vi "IMURead.vi"(0 "AdaIMUDevRef":T4={"DevStatus"={"status"=FALSE, "code"=0, "source"=""}, "Gyro Address"=0, "Gyro Range"=0, "Mean Rates"={"Xmo"=0.0, "Ymo"=0.0, "Zmo"=0.0}, "StdDev Rates"={"Xsdo"=0.0, "Ysdo"=0.0, "Zsdo"=0.0}, "Fast"=FALSE, "Reset"=FALSE, "Accel Address"=0, "Accel Range"=0, "Accel Scale"={"Xscale"=0.0, "Yscale"=0.0, "Zscale"=0.0}, "Mag Address"=0, "Mag Range"=0, "G Sense"=FALSE, "A Sense"=FALSE, "M Sense"=FALSE, "Accel Offset"={"Xzero"=0.0, "Yzero"=0.0, "Zzero"=0.0}, "Motion Thresh"=0.0, "Mag Scale"={"Xscale"=1.0, "Yscale"=1.0, "Zscale"=1.0}, "Mag Offset"={"Xzero"=1.0, "Yzero"=1.0, "Zzero"=1.0}, "I2C Bus"=enum."I2C On-Board", "Handle"=0, "Anomaly Thresh"=0.0, "Local Mag"=0.0}, 11 "error in":errorcluster) -> (4 "AdaIMUDevRef Out":T4={"DevStatus"={"status"=FALSE, "code"=0, "source"=""}, "Gyro Address"=0, "Gyro Range"=0, "Mean Rates"={"Xmo"=0.0, "Ymo"=0.0, "Zmo"=0.0}, "StdDev Rates"={"Xsdo"=0.0, "Ysdo"=0.0, "Zsdo"=0.0}, "Fast"=FALSE, "Reset"=FALSE, "Accel Address"=0, "Accel Range"=0, "Accel Scale"={"Xscale"=0.0, "Yscale"=0.0, "Zscale"=0.0}, "Mag Address"=0, "Mag Range"=0, "G Sense"=FALSE, "A Sense"=FALSE, "M Sense"=FALSE, "Accel Offset"={"Xzero"=0.0, "Yzero"=0.0, "Zzero"=0.0}, "Motion Thresh"=0.0, "Mag Scale"={"Xscale"=1.0, "Yscale"=1.0, "Zscale"=1.0}, "Mag Offset"={"Xzero"=1.0, "Yzero"=1.0, "Zzero"=1.0}, "I2C Bus"=enum."I2C On-Board", "Handle"=0, "Anomaly Thresh"=0.0, "Local Mag"=0.0}, 6 "Gyro":T3, 8 "Accel":T1={"Xaccel"=0.0, "Yaccel"=0.0, "Zaccel"=0.0, "Motion"=FALSE, "Threshold"=0.04, "FreeFall"=FALSE}, 10 "Mag":T2, 15 "error out":errorcluster)   [LabVIEW 2015]
uses:
  IMUDevRef.ctl
  <vilib>/Rock Robotics/SystemInterfaces/i2clib/i2c_bus.ctl
  Gyro.ctl
  Mag.ctl
  Accel.ctl
  <vilib>/Rock Robotics/WPI/I2C/WPI_I2CDevRef.ctl
panel:
  # "When Sensor oriented with positive X-axis\npointing forward, and positive Y-axis\npointing left, and positive Z axis pointing up :\n\nRoll is rotation about X-axis, clockwise roll,\n(looking in + X direction), is positive.\n\nPitch is rotation about Y-axis, clockwise pitch\n(looking in + Y direction), is positive.\n\nYaw is rotation about Z-axis, clockwise yaw\n(looking in + Z direction), is positive."
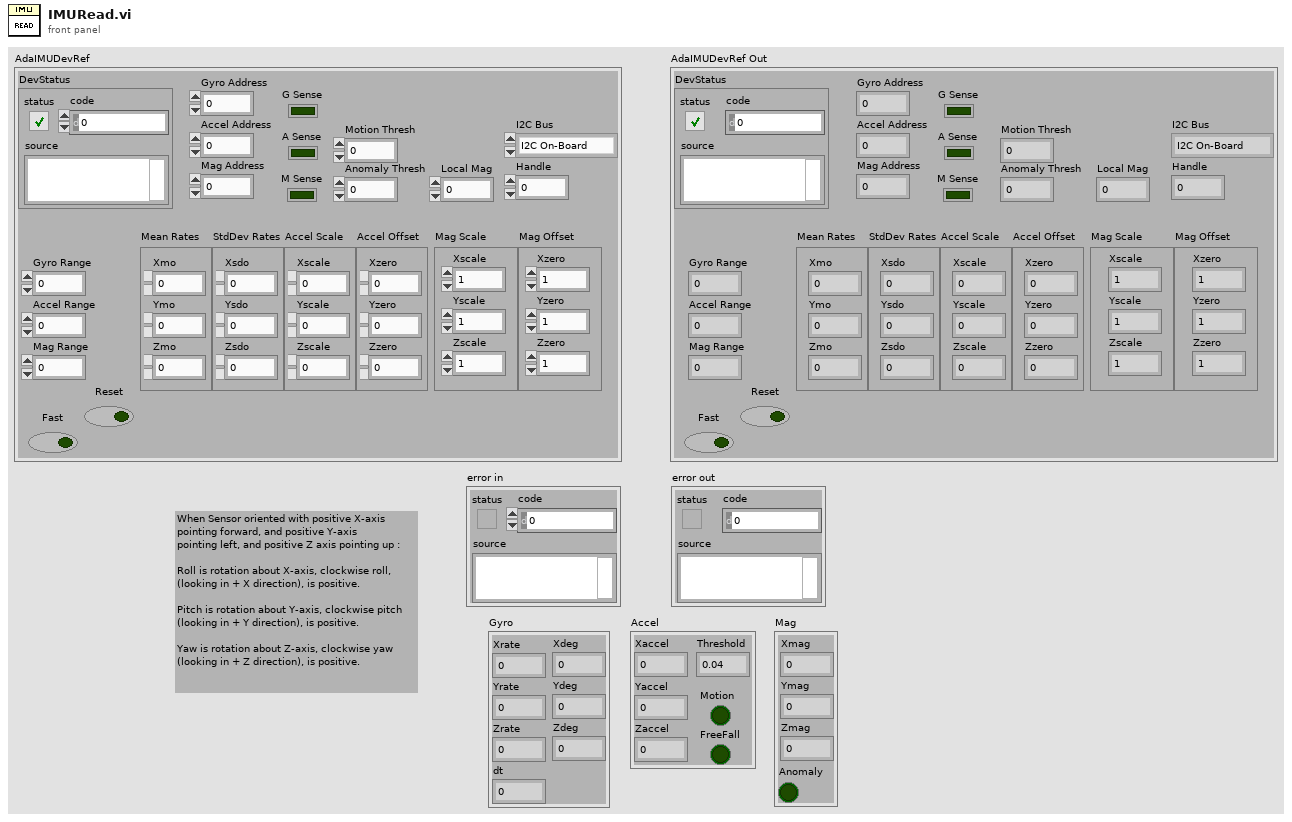
[diagram p1: front panel]
types:
  T1 = typedef "Accel.ctl" = cluster{"Xaccel":dbl, "Yaccel":dbl, "Zaccel":dbl, "Motion":bool, "Threshold":dbl, "FreeFall":bool}
  T2 = typedef "Mag.ctl" = cluster{"Xmag":dbl, "Ymag":dbl, "Zmag":dbl, "Anomaly":bool}
  T3 = typedef "Gyro.ctl" = cluster{"Xrate":dbl, "Yrate":dbl, "Zrate":dbl, "Xdeg":dbl, "Ydeg":dbl, "Zdeg":dbl, "dt":dbl}
  T4 = typedef "IMUDevRef.ctl" = cluster{"DevStatus":errorcluster, "Gyro Address":u8, "Gyro Range":u8, "Mean Rates":cluster{"Xmo":dbl, "Ymo":dbl, "Zmo":dbl}, "StdDev Rates":cluster{"Xsdo":dbl, "Ysdo":dbl, "Zsdo":dbl}, "Fast":bool, "Reset":bool, "Accel Address":u8, "Accel Range":u8, "Accel Scale":cluster{"Xscale":dbl, "Yscale":dbl, "Zscale":dbl}, "Mag Address":u8, "Mag Range":u8, "G Sense":bool, "A Sense":bool, "M Sense":bool, "Accel Offset":cluster{"Xzero":dbl, "Yzero":dbl, "Zzero":dbl}, "Motion Thresh":dbl, "Mag Scale":cluster{"Xscale":dbl, "Yscale":dbl, "Zscale":dbl}, "Mag Offset":cluster{"Xzero":dbl, "Yzero":dbl, "Zzero":dbl}, "I2C Bus":T5, "Handle":i32, "Anomaly Thresh":dbl, "Local Mag":dbl}
  T5 = typedef "i2c_bus.ctl" = enum16{"I2C On-Board", "I2C MXP", "Invalid"}
  T6 = typedef "WPI_I2CDevRef.ctl" = cluster{"DevStatus":errorcluster, "Device Address":u8, "Handle":i32, "I2C Bus":T5}
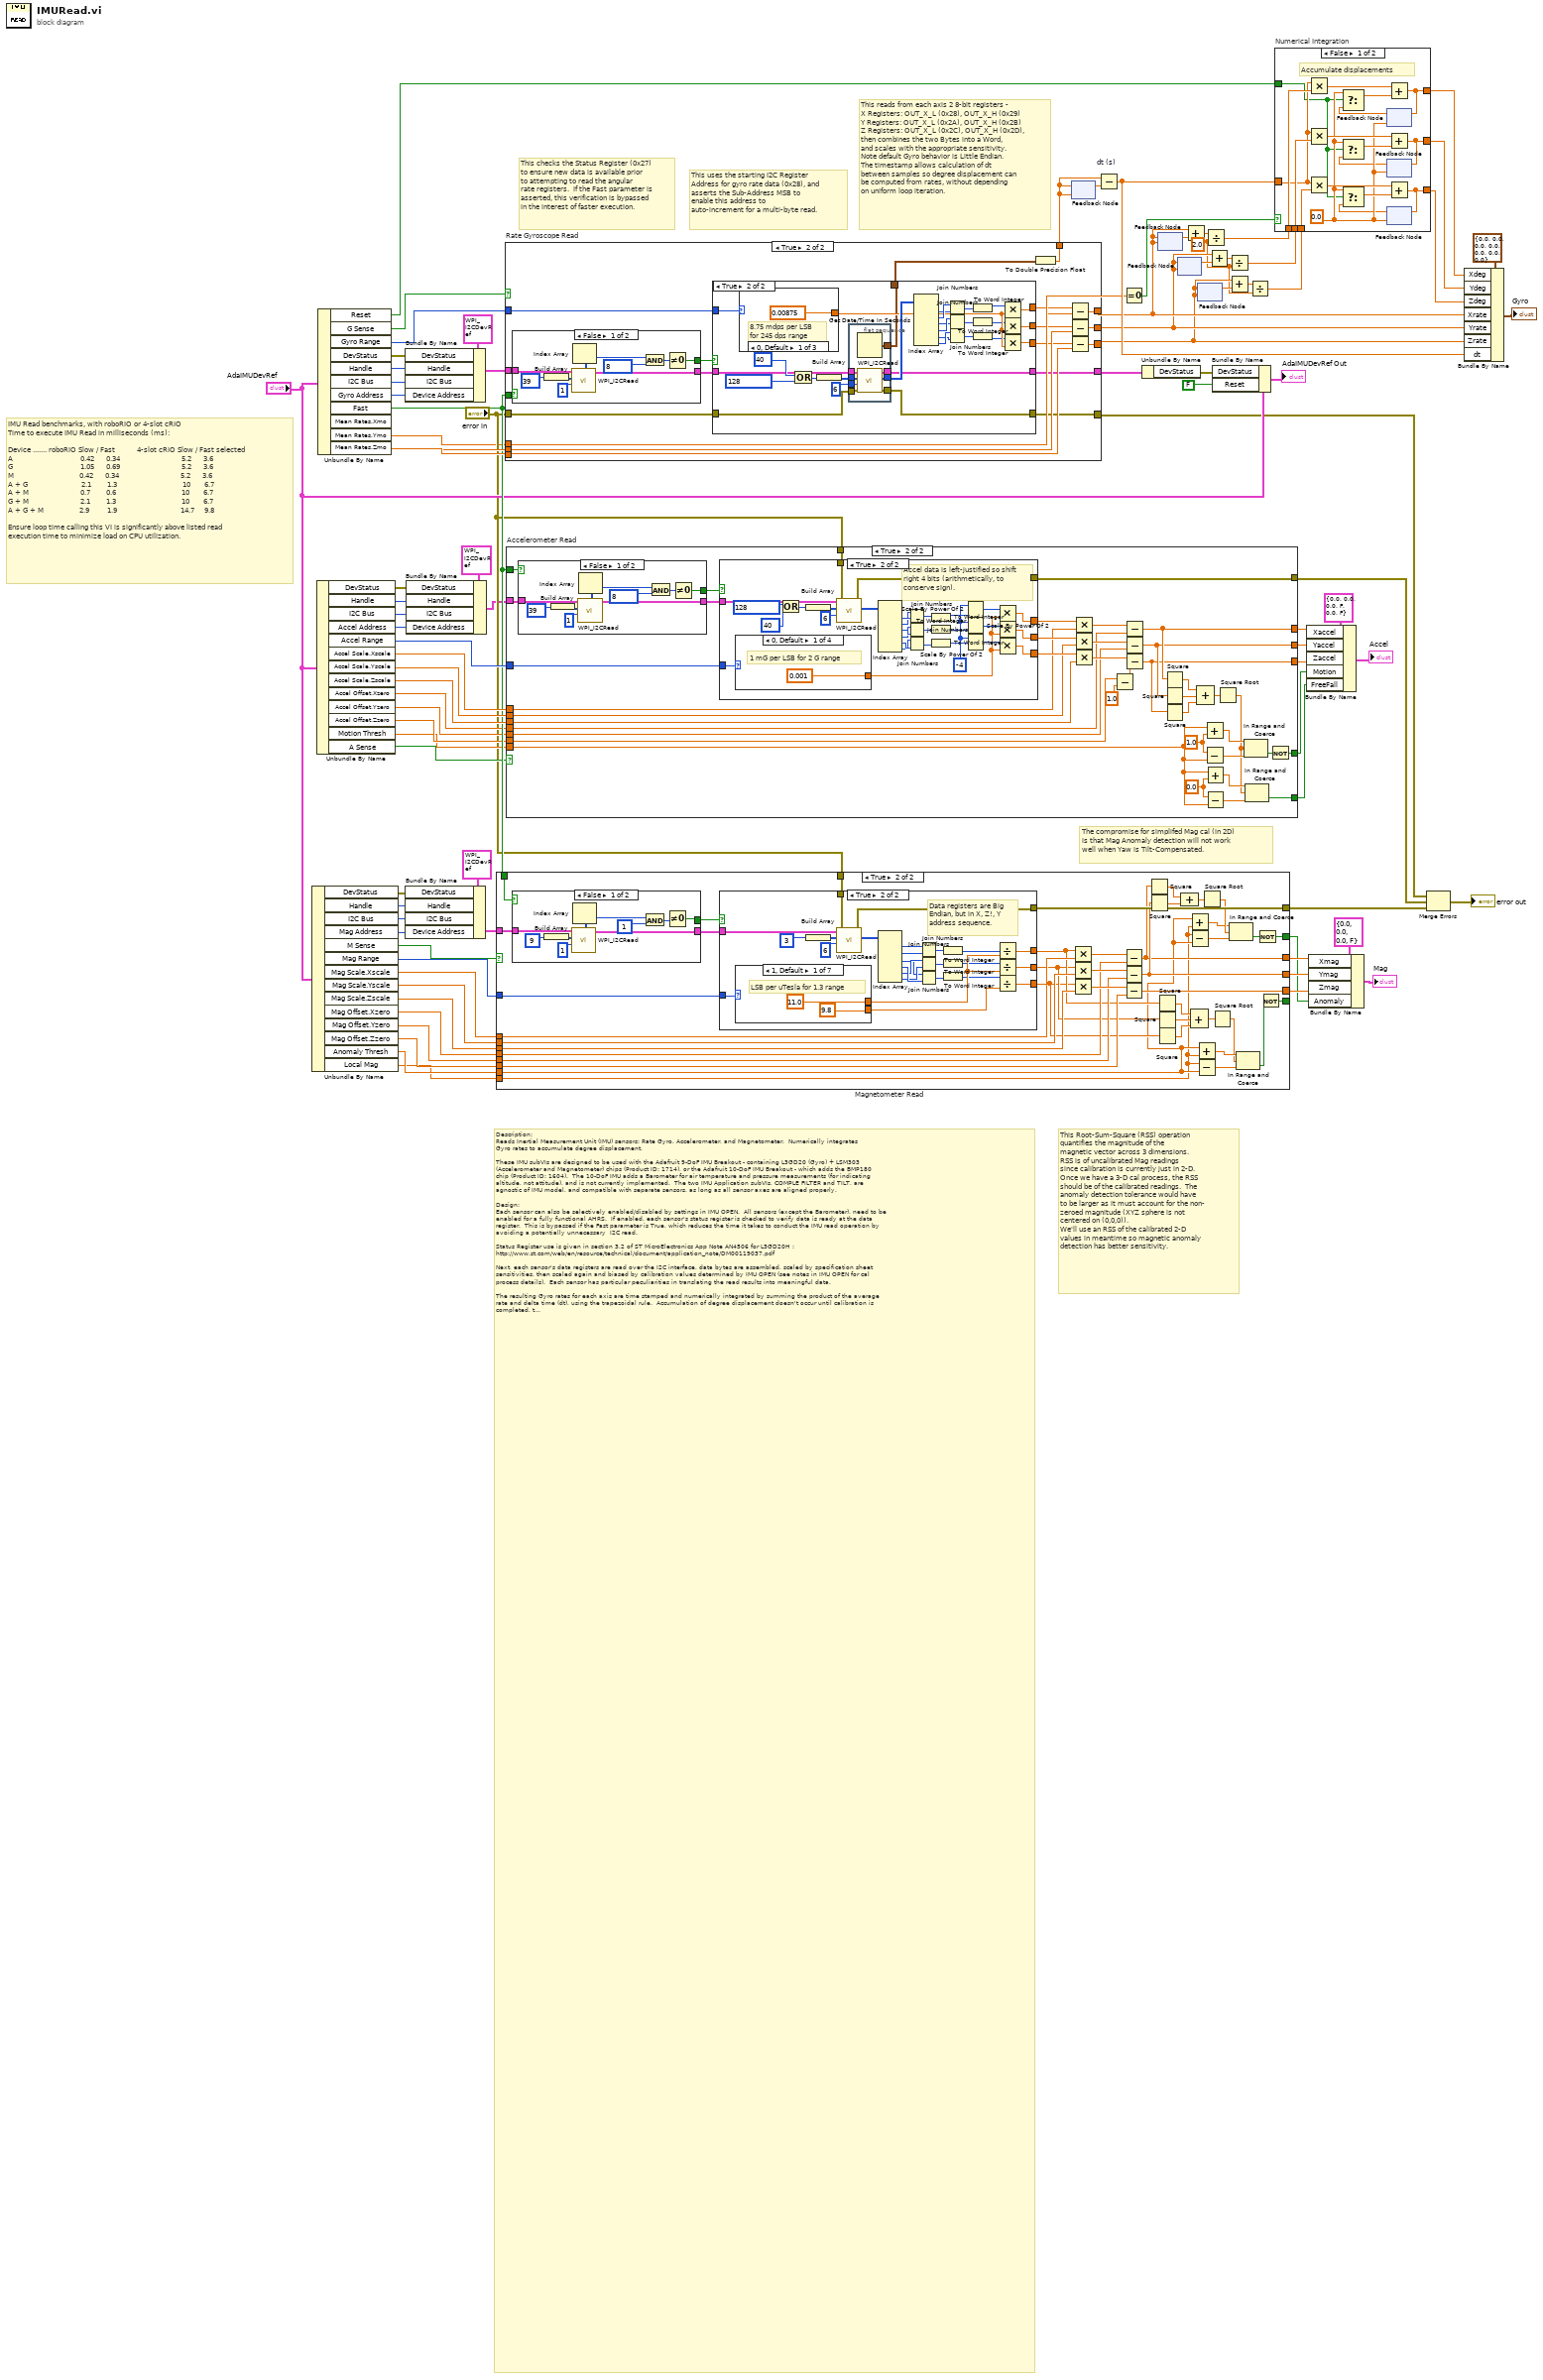
[diagram p0: block diagram]
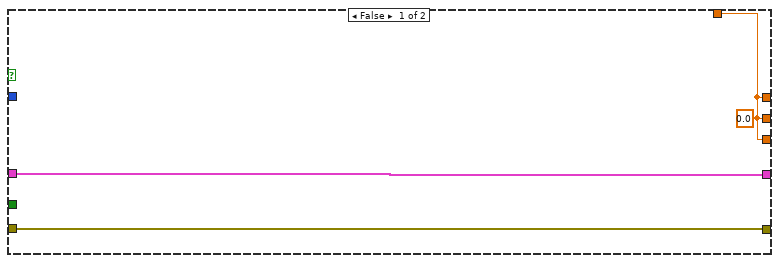
[diagram p2: hidden frame]
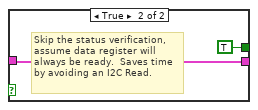
[diagram p3: hidden frame]
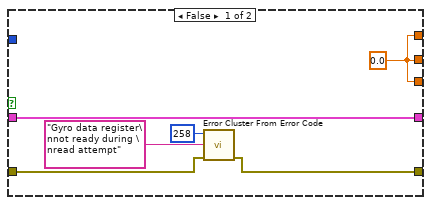
[diagram p4: hidden frame]
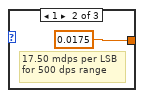
[diagram p5: hidden frame]
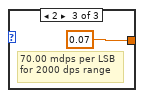
[diagram p6: hidden frame]
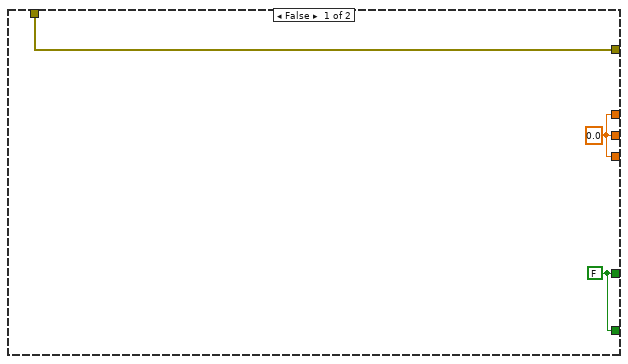
[diagram p7: hidden frame]
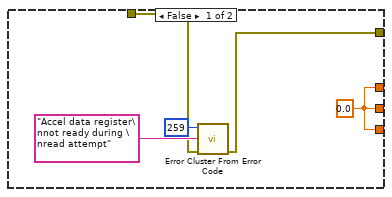
[diagram p8: hidden frame]
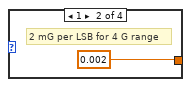
[diagram p9: hidden frame]
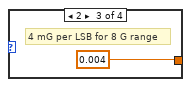
[diagram p10: hidden frame]
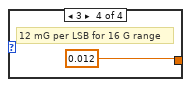
[diagram p11: hidden frame]
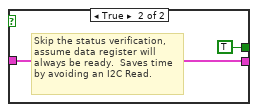
[diagram p12: hidden frame]
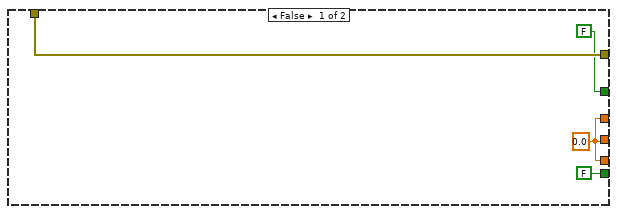
[diagram p13: hidden frame]
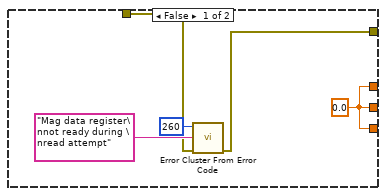
[diagram p14: hidden frame]
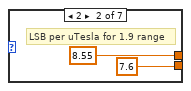
[diagram p15: hidden frame]
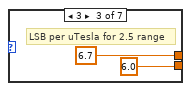
[diagram p16: hidden frame]
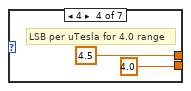
[diagram p17: hidden frame]
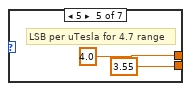
[diagram p18: hidden frame]
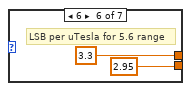
[diagram p19: hidden frame]
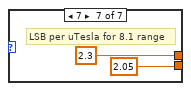
[diagram p20: hidden frame]
diagram:
  w22 = 2.0 ("y")
  # "The compromise for simplifed Mag cal (in 2D)\nis that Mag Anomaly detection will not work\nwell when Yaw is Tilt-Compensated."
  # "This Root-Sum-Square (RSS) operation\nquantifies the magnitude of the\nmagnetic vector across 3 dimensions.\nRSS is of uncalibrated Mag readings\nsince calibration is currently just in 2-D.\nOnce we have a 3-D cal process, the RSS\nshould be of the calibrated readings.  The\nanomaly detection tolerance would have \nto be larger as it must account for the non-\nzeroed magnitude (XYZ sphere is not\ncentered on (0,0,0)). \nWe'll use an RSS of the calibrated 2-D\nvalues in meantime so magnetic anomaly\ndetection has better sensitivity."
  # "Description:\nReads Inertial Measurement Unit (IMU) sensors: Rate Gyro, Accelerometer, and Magnetometer.  Numerically integrates\nGyro rates to accumulate degree displacement.\n\nThese IMU subVIs are designed to be used with the Adafruit 9-DoF IMU Breakout - containing L3GD20 (Gyro) + LSM303 \n(Accelerometer and Magnetometer) chips (Product ID: 1714), or the Adafruit 10-DoF IMU Breakout - which adds the BMP180\nchip (Product ID: 1604).  The 10-DoF IMU adds a Barometer for air temperature and pressure measurements (for indicating\naltitude, not attitude), and is not currently implemented.  The two IMU Application subVIs, COMPLE FILTER and TILT, are\nagnostic of IMU model, and compatible with separate sensors, as long as all sensor axes are aligned properly.\n\nDesign:\nEach sensor can also be selectively enabled/disabled by settings in IMU OPEN.  All sensors (except the Barometer), need to be\nenabled for a fully functional AHRS.  If enabled, each sensor's status register is checked to verify data is ready at the data\nregister.  This is bypassed if the Fast parameter is True, which reduces the time it takes to conduct the IMU read operation by\navoiding a potentially unnecessary  I2C read.  \n\nStatus Register use is given in section 3.2 of ST MicroElectronics App Note AN4506 for L3GD20H : \nhttp://www.st.com/web/en/resource/technical/document/application_note/DM00119037.pdf\n\nNext, each sensor's data registers are read over the I2C interface, data bytes are assembled, scaled by specification sheet\nsensitivities, then scaled again and biased by calibration values determined by IMU OPEN (see notes in IMU OPEN for cal\nprocess details).  Each sensor has particular peculiarities in translating the read results into meaningful data.\n\nThe resulting Gyro rates for each axis are time stamped and numerically integrated by summing the product of the average\nrate and delta time (dt), using the trapezoidal rule.  Accumulation of degree displacement doesn't occur until calibration is\ncompleted, to allow IMU OPEN to make use of IMU READ for the cal process (code reuse).  Resetting the degree displacements\nto zero is accomplished by IMU RESET generating a flag via the IMU DevRef cluster, requiring the 'reset' signal to always be\nupstream of the IMU READ, which is then cleared here.  The native data register sequence is Little Endian - review this term and\nits relationship to Gulliver’s Travels by Jonathan Swift for insight on reference.  Rates, Degrees, and dt are provided in a Gyro\noutput cluster.\n\nAlthough each sensor shares the basic design of storing their measurements across two one-byte registers, the Accelerometer\ndata registers are left-justified (and Little Endian), with the lowest 4 bits of the lowest byte containing no data.  (Gyro and\nMagnetometer data registers are both right-justified.)  Presumably the left-justification provides a means to read the Accel\nfaster by reading only the upper byte, should one not require the additional precision contained in the lower byte.  Since we\nare using both bytes for maximum precision, the concatenation of the two bytes must be right-shifted by 4 bits.  This must be\ndone with an arithmetic shift, rather than a logical shift, to preserve the sign bit encoded within the twos-complement storage\nformat.  \n\nMovement and Free Fall are detected by comparing the root-sum-square of the 3 axes to value 1 (G) for movement\ndetection and 0 (G) for Free Fall using a common Threshold value as tolerance for the comparison.  A future improvement is to\ntake advantage of the Accelerometer's on-board Free Fall detection capability, i.e., moving the detection into hardware for\nsuperior response, which could be sensed with a DIO port. Each calibrated axis reading is provided in a Accel output cluster\nalong with Movement and Free Fall Booleans.\n\nThe Magnetometer data registers are Big Endian, but are peculiar in that the register address sequence is X-Z-Y instead of X-Y-Z.\nThis is non-obvious and was clearly done to simply torture me.  Magnetic Anomalies are detected by comparing the\nroot-sum-square of the X and Y axes (2-D) to the horizontal magnitude of the local Earth field.  One can use the value calculated\nduring the magnetic calibration process, which should be consistent with data available at the National Geophysical Data Center\n\n(NOAA/NGDC at http://www.ngdc.noaa.gov/geomag-web/?useFullSite=true#igrfwmm)\n\n... input USA zip code or city/country, select Get Lat/Long then Calculate, and note \"Horizontal Intensity\", expressing this in\nmicroTeslas (not nanoTeslas as NOAA displays).  An Anomaly Threshold value is used as tolerance for the comparison.  Each\ncalibrated axis reading is provided in a Mag output cluster along with a Magnetic Anomaly Boolean.\n\nInputs:\nADAIMUDEVREF - Device Reference containing IMU configuration data.  Sensor enable condition, range, I2C address, and\n                                calibration parameters are stored here.\nOutputs:\nADAIMUDEVREF OUT - Device Reference containing IMU configuration data.  Gyro reset is cleared as each IMU READ completes.\nGYRO - Cluster containing rate and displacements for each axis with delta time since last data point.\nACCEL - Cluster containing, for each axis, calibrated acceleration measurement with movement/free fall indications and threshold.\nMAG - Cluster containing, for each axis, calibrated magnetic measurement with magnetic anomaly indication.\nANOMALY - Boolean indicating that a magnetic anomaly is detected.\n\nFuture Improvements:\nMove freefall into interrupt/DIO, Auto ranging, FPGA numerical integration or Simpson's Rule to improve off-FPGA numerical\nintegration, SPI interface for potentially faster read response.\n\n\nVI Properties:\nExecution Reentrancy is set to Non Reentrant Execution\n\nImplementation:\nThis design performs numerical integration off-FPGA for the Digital Gyro (unlike the Analog Gyro subVIs, which typically utilize\nthe FPGA to perform accumulation for superior speed resulting in less integration error).   Testing indicates this off-FPGA\napproach may be adequate for FRC application, however, it is important to ensure the code runs without any timing issues.\nThis is why a Timed Loop is recommended for the IMU Read within Periodic Tasks (executes at a higher priority).  Non-uniformity\nin read iteration is mitigated by design, as each dt is uniquely calculated by time stamping each read event.  This means that while\nsome variation in timing can be tolerated (the occasional late iteration), excessively long durations (periods) between successive\nreads will fail to capture the actual rate profile as it changes resulting in integration error.  \n\nIn short, use a Timed Loop structure to iterate IMU READs, and set the loop period for a relatively fast iteration (<75 ms).  Shorter\nperiods provide improved accuracy of degree displacements, however setting this too short can impact the execution of your\nremaining code (especially when using Timed Loops).  One way of determining an optimized period is to set it while monitoring\nthe \"Finished Late?\" Loop parameter, ensuring this value stays False.   It helps if the CPU Utilization remains low (<75%), which\ncan be monitored with the RT Get CPU Loads subVI (Real Time menu).  Study LabVIEW determinism for additional insight.\n\nIMU Read benchmarks, with roboRIO or 4-slot cRIO\nTime to execute IMU Read in milliseconds (ms):\n\nSensor ....... roboRIO Slow / Fast           4-slot cRIO Slow / Fast selected\nA                                  0.42      0.34                               5.2      3.6\nG                                  1.05      0.69                               5.2      3.6\nM                                 0.42      0.34                               5.2      3.6\nA + G                           2.1        1.3                                 10       6.7\nA + M                          0.7        0.6                                 10       6.7\nG + M                          2.1        1.3                                 10       6.7\nA + G + M                  2.9         1.9                                14.7     9.8\n\n(\"Slow\" is when Fast is deasserted).\n\nEnsure loop time calling this VI is significantly above listed read execution time to minimize load on CPU utilization.\n\n----- The RoboBees FRC Team 836! -----  You too can conquer inertia!! ... consider a career in STEM!"
  # "IMU Read benchmarks, with roboRIO or 4-slot cRIO\nTime to execute IMU Read in milliseconds (ms):\n\nDevice ....... roboRIO Slow / Fast           4-slot cRIO Slow / Fast selected\nA                                  0.42      0.34                               5.2      3.6\nG                                  1.05      0.69                               5.2      3.6\nM                                 0.42      0.34                               5.2      3.6\nA + G                           2.1        1.3                                 10       6.7\nA + M                          0.7        0.6                                 10       6.7\nG + M                          2.1        1.3                                 10       6.7\nA + G + M                  2.9         1.9                                14.7     9.8\n\nEnsure loop time calling this VI is significantly above listed read\nexecution time to minimize load on CPU utilization."
  # "This reads from each axis 2 8-bit registers - \nX Registers: OUT_X_L (0x28), OUT_X_H (0x29)\nY Registers: OUT_X_L (0x2A), OUT_X_H (0x2B)\nZ Registers: OUT_X_L (0x2C), OUT_X_H (0x2D),\nthen combines the two Bytes into a Word,\nand scales with the appropriate sensitivity.\nNote default Gyro behavior is Little Endian.\nThe timestamp allows calculation of dt\nbetween samples so degree displacement can\nbe computed from rates, without depending\non uniform loop iteration."
  # "This checks the Status Register (0x27)\nto ensure new data is available prior\nto attempting to read the angular\nrate registers.  If the Fast parameter is\nasserted, this verification is bypassed\nin the interest of faster execution."
  # "This uses the starting I2C Register\nAddress for gyro rate data (0x28), and\nasserts the Sub-Address MSB to\nenable this address to \nauto-increment for a multi-byte read."
  n1 = Unbundle By Name("AdaIMUDevRef") -> ("DevStatus"=w66:errorcluster, "Handle"=w11:i32, "I2C Bus"=w10:T5, "Mag Address"=w12:u8, "M Sense"=w48:bool, "Mag Range"=w49:u8, "Mag Scale.Xscale"=w8:dbl, "Mag Scale.Yscale"=w33:dbl, "Mag Scale.Zscale"=w36:dbl, "Mag Offset.Xzero"=w35:dbl, "Mag Offset.Yzero"=w34:dbl, "Mag Offset.Zzero"=w9:dbl, "Anomaly Thresh"=w7:dbl, "Local Mag"=w6:dbl)
  n2 = Unbundle By Name("AdaIMUDevRef") -> ("DevStatus"=w74:errorcluster, "Handle"=w13:i32, "I2C Bus"=w14:T5, "Accel Address"=w15:u8, "Accel Range"=w73:u8, "Accel Scale.Xscale"=w72:dbl, "Accel Scale.Yscale"=w71:dbl, "Accel Scale.Zscale"=w70:dbl, "Accel Offset.Xzero"=w58:dbl, "Accel Offset.Yzero"=w57:dbl, "Accel Offset.Zzero"=w56:dbl, "Motion Thresh"=w50:dbl, "A Sense"=w47:bool)
  n3 = Unbundle By Name("AdaIMUDevRef") -> ("Reset"=w44:bool, "G Sense"=w43:bool, "Gyro Range"=w69:u8, "DevStatus"=w76:errorcluster, "Handle"=w18:i32, "I2C Bus"=w17:T5, "Gyro Address"=w16:u8, "Fast"=w65:bool, "Mean Rates.Xmo"=w19:dbl, "Mean Rates.Ymo"=w88:dbl, "Mean Rates.Zmo"=w89:dbl)
  n4 = Bundle By Name(cluster=T6 {"DevStatus"={"status"=FALSE, "code"=0, "source"=""}, "Device Address"=107, "Handle"=28, "I2C Bus"=enum."I2C On-Board"} ("I2CDevRef 2"), "DevStatus"=w76, "Handle"=w18, "I2C Bus"=w17, "Device Address"=w16) -> (w68:T6)
  n5 = Bundle By Name(cluster=T6 {"DevStatus"={"status"=FALSE, "code"=0, "source"=""}, "Device Address"=107, "Handle"=28, "I2C Bus"=enum."I2C On-Board"} ("I2CDevRef 2"), "DevStatus"=w66, "Handle"=w11, "I2C Bus"=w10, "Device Address"=w12) -> (w67:T6)
  n6 = Bundle By Name(cluster=T6 {"DevStatus"={"status"=FALSE, "code"=0, "source"=""}, "Device Address"=107, "Handle"=28, "I2C Bus"=enum."I2C On-Board"} ("I2CDevRef 2"), "DevStatus"=w74, "Handle"=w13, "I2C Bus"=w14, "Device Address"=w15) -> (w5:T6)
  n7 = case "Magnetometer Read" shown="True" w48 {
    tunnel: w67 -> [_ w134]
    tunnel: w49 -> [_ w131]
    tunnel: "error in" -> [w92 w130]
    tunnel: [w92 w129] -> w38
    tunnel: w65 -> [_ w128]
    tunnel: [w93 w97] -> w62
    tunnel: [w93 w98] -> w61
    tunnel: [w93 w112] -> w60
    tunnel: w8 -> [_ w124]
    tunnel: w33 -> [_ w123]
    tunnel: w36 -> [_ w122]
    tunnel: w35 -> [_ w121]
    tunnel: w34 -> [_ w120]
    tunnel: w9 -> [_ w119]
    tunnel: [FALSE w107] -> _
    tunnel: w7 -> [_ w96]
    tunnel: w6 -> [_ w95]
    tunnel: [FALSE w94] -> w1
    frame False {
      w93 = 0.0
    }
    frame True {
      n8 = case shown="False" w128 {
        tunnel: w134 -> [w179 w189]
        tunnel: [w184 w189] -> w132
        tunnel: [w180 TRUE] -> w133
        frame False {
          n9 = Build Array(u8 9 ("Data To Send")) -> (w188:u8[])
          n10 = call <vilib>:"WPI_I2CRead.vi"("I2CBytesToRead"=u8 1, "I2CRegister"=w188, "I2CDevRef"=w179) -> ("Data Out"=w185:u8[], "I2CDevRef"=w184:T6)  [unwired: 6 in, 1 out]
          n11 = Index Array(array=w185) -> (element=w182:u8)  [unwired: 1 in]
          n12 = And(x=w182, y=u8 1 ("Data To Send")) -> (x .and. y?=w181:u8)
          n13 = Not Equal To 0?(x=w181) -> (x != 0?=w180:bool)
        }
        frame True {
          # "Skip the status verification,\nassume data register will\nalways be ready.  Saves time\nby avoiding an I2C Read."
        }
      }
      n14 = case shown="True" w133 {
        tunnel: [w139 w157] -> w110
        tunnel: [w139 w156] -> w109
        tunnel: [w139 w155] -> w108
        tunnel: w131 -> [_ w154]
        tunnel: w132 -> [_ w153]
        tunnel: w130 -> [w136 w152]
        tunnel: [w135 w151] -> w129
        frame False {
          w139 = 0.0
          n15 = call <vilib>:"Error Cluster From Error Code.vi"("error in (no error)"=w136, "error message (\"\")"="Mag data register\nnot ready during \nread attempt" ("error message (\"\")"), "error code (0)"=260) -> ("error out"=w135:errorcluster)  [unwired: 6 in]
        }
        frame True {
          # "Data registers are Big\nEndian, but in X, Z!, Y\naddress sequence."
          n16 = case shown="1, Default" w154 {
            tunnel: [11.0 ("y") 8.55 ("y") 6.7 ("y") 4.5 ("y") 4.0 ("y") 3.3 ("y") 2.3 ("y")] -> w158
            tunnel: [9.8 ("y") 7.6 ("y") 6.0 ("y") 4.0 ("y") 3.55 ("y") 2.95 ("y") 2.05 ("y")] -> w144
            frame 1, Default {
              # "LSB per uTesla for 1.3 range"
            }
            frame 2 {
              # "LSB per uTesla for 1.9 range"
            }
            frame 3 {
              # "LSB per uTesla for 2.5 range"
            }
            frame 4 {
              # "LSB per uTesla for 4.0 range"
            }
            frame 5 {
              # "LSB per uTesla for 4.7 range"
            }
            frame 6 {
              # "LSB per uTesla for 5.6 range"
            }
            frame 7 {
              # "LSB per uTesla for 8.1 range"
            }
          }
          n17 = Build Array(u8 3 ("Data To Send")) -> (w161:u8[])
          n18 = call <vilib>:"WPI_I2CRead.vi"("error in (no error)"=w152, "I2CBytesToRead"=u8 6, "I2CRegister"=w161, "I2CDevRef"=w153) -> ("error out"=w151:errorcluster, "Data Out"=w163:u8[])  [unwired: 5 in, 1 out]
          n19 = Index Array(array=w163) -> (element #1=w149:u8, element #2=w148:u8, element #3=w140:u8, element #4=w143:u8, element #5=w142:u8, element #6=w141:u8)  [unwired: 6 in]
          n20 = Join Numbers(hi=w149, lo=w148) -> ((hi.lo)=w162:u16)
          n21 = Join Numbers(hi=w142, lo=w141) -> ((hi.lo)=w159:u16)
          n22 = Join Numbers(hi=w140, lo=w143) -> ((hi.lo)=w160:u16)
          n23 = To Word Integer(number=w162) -> (16bit integer=w147:i16)
          n24 = To Word Integer(number=w159) -> (16bit integer=w146:i16)
          n25 = To Word Integer(number=w160) -> (16bit integer=w145:i16)
          n26 = Divide(x=w147, y=w158) -> (x/y=w157:dbl)
          n27 = Divide(x=w146, y=w158) -> (x/y=w156:dbl)
          n28 = Divide(x=w145, y=w144) -> (x/y=w155:dbl)
        }
      }
      n29 = Multiply(x=w110, y=w124) -> (x*y=w125:dbl)
      n30 = Multiply(x=w109, y=w123) -> (x*y=w126:dbl)
      n31 = Multiply(x=w108, y=w122) -> (x*y=w127:dbl)
      n32 = Subtract(x=w125, y=w121) -> (x-y=w97:dbl)
      n33 = Subtract(x=w126, y=w120) -> (x-y=w98:dbl)
      n34 = Subtract(x=w127, y=w119) -> (x-y=w112:dbl)
      n35 = Square(x=w97) -> (x^2=w103:dbl)
      n36 = Square(x=w98) -> (x^2=w102:dbl)
      n37 = Square(x=w110) -> (x^2=w113:dbl)
      n38 = Square(x=w109) -> (x^2=w114:dbl)
      n39 = Square(x=w108) -> (x^2=w115:dbl)
      n40 = Compound Arithmetic op=ADD(w103, w102) -> (w101:dbl)
      n41 = Add(x=w96, y=w95) -> (x+y=w99:dbl)
      n42 = Subtract(x=w95, y=w96) -> (x-y=w100:dbl)
      n43 = Compound Arithmetic op=ADD(w113, w114, w115) -> (w116:dbl)
      n44 = Add(x=w96, y=w95) -> (x+y=w118:dbl)
      n45 = Subtract(x=w95, y=w96) -> (x-y=w117:dbl)
      n46 = Square Root(x=w101) -> (sqrt(x)=w104:dbl)
      n47 = Square Root(x=w116) -> (sqrt(x)=w111:dbl)
      n48 = In Range and Coerce(upper limit=w99, x=w104, lower limit=w100) -> (In Range?=w105:bool)  [unwired: 1 out]
      n49 = In Range and Coerce(upper limit=w118, x=w111, lower limit=w117) -> (In Range?=w106:bool)  [unwired: 1 out]
      n50 = Not(x=w105) -> (.not. x?=w94:bool)
      n51 = Not(x=w106) -> (.not. x?=w107:bool)
    }
  }
  n52 = case "Rate Gyroscope Read" shown="True" w43 {
    tunnel: w89 -> [_ w212]
    tunnel: w88 -> [_ w211]
    tunnel: w19 -> [_ w210]
    tunnel: [w193 w206] -> w23
    tunnel: [w193 w204] -> w78
    tunnel: w69 -> [_ w201]
    tunnel: w68 -> [w192 w200]
    tunnel: [w191 w199] -> w42
    tunnel: w65 -> [_ w198]
    tunnel: [w193 w197] -> w29
    tunnel: [w193 w196] -> w24
    tunnel: [w192 w195] -> w46
    tunnel: "error in" -> [w191 w194]
    frame False {
      w193 = 0.0
    }
    frame True {
      n53 = case shown="False" w198 {
        tunnel: w200 -> [w213 w224]
        tunnel: [w218 w224] -> w203
        tunnel: [w215 TRUE] -> w202
        frame False {
          n54 = Build Array(u8 39 ("Data To Send")) -> (w222:u8[])
          n55 = call <vilib>:"WPI_I2CRead.vi"("I2CBytesToRead"=u8 1, "I2CRegister"=w222, "I2CDevRef"=w213) -> ("Data Out"=w219:u8[], "I2CDevRef"=w218:T6)  [unwired: 6 in, 1 out]
          n56 = Index Array(array=w219) -> (element=w216:u8)  [unwired: 1 in]
          n57 = And(x=w216, y=u8 8 ("Data To Send")) -> (x .and. y?=w217:u8)
          n58 = Not Equal To 0?(x=w217) -> (x != 0?=w215:bool)
        }
        frame True {
          # "Skip the status verification,\nassume data register will\nalways be ready.  Saves time\nby avoiding an I2C Read."
        }
      }
      n59 = case shown="True" w202 {
        tunnel: [w226 w258] -> w209
        tunnel: w194 -> [w230 w257]
        tunnel: [w229 w256] -> w199
        tunnel: w203 -> [w225 w247]
        tunnel: [w226 w244] -> w208
        tunnel: [w226 w243] -> w207
        tunnel: w201 -> [_ w240]
        tunnel: [_ w238] -> w205
        tunnel: [w225 w231] -> w195
        frame False {
          w226 = 0.0
          n60 = call <vilib>:"Error Cluster From Error Code.vi"("error in (no error)"=w230, "error message (\"\")"="Gyro data register\nnot ready during \nread attempt" ("error message (\"\")"), "error code (0)"=258) -> ("error out"=w229:errorcluster)  [unwired: 6 in]
        }
        frame True {
          n61 = case shown="0, Default" w240 {
            tunnel: [0.00875 ("y") 0.0175 ("y") 0.07 ("y")] -> w239
            frame 0, Default {
              # "8.75 mdps per LSB\nfor 245 dps range"
            }
            frame 1 {
              # "17.50 mdps per LSB\nfor 500 dps range"
            }
            frame 2 {
              # "70.00 mdps per LSB\nfor 2000 dps range"
            }
          }
          n62 = Or(x=u8 40 ("Data To Send"), y=u8 128 ("Data To Send")) -> (x .or. y?=w252:u8)
          n63 = Build Array(w252) -> (w254:u8[])
          n64 = flat-sequence {
            tunnel: w257 -> [w266]
            tunnel: [w265] -> w256
            tunnel: [w264] -> w255
            tunnel: w254 -> [w263]
            tunnel: u8 6 ("I2CBytesToRead") -> [w262]
            tunnel: w247 -> [w261]
            tunnel: [w260] -> w238
            tunnel: [w259] -> w231
            frame #0 {
              n65 = Get Date/Time In Seconds() -> (seconds since 1Jan1904=w260:timestamp)
              n66 = call <vilib>:"WPI_I2CRead.vi"("error in (no error)"=w266, "I2CBytesToRead"=w262, "I2CRegister"=w263, "I2CDevRef"=w261) -> ("error out"=w265:errorcluster, "Data Out"=w264:u8[], "I2CDevRef"=w259:T6)  [unwired: 5 in]
            }
          }
          n67 = Index Array(array=w255) -> (element #1=w248:u8, element #2=w249:u8, element #3=w241:u8, element #4=w242:u8, element #5=w245:u8, element #6=w246:u8)  [unwired: 6 in]
          n68 = Join Numbers(hi=w249, lo=w248) -> ((hi.lo)=w237:u16)
          n69 = Join Numbers(hi=w242, lo=w241) -> ((hi.lo)=w235:u16)
          n70 = Join Numbers(hi=w246, lo=w245) -> ((hi.lo)=w234:u16)
          n71 = To Word Integer(number=w237) -> (16bit integer=w236:i16)
          n72 = To Word Integer(number=w235) -> (16bit integer=w233:i16)
          n73 = To Word Integer(number=w234) -> (16bit integer=w232:i16)
          n74 = Multiply(x=w236, y=w239) -> (x*y=w258:dbl)
          n75 = Multiply(x=w233, y=w239) -> (x*y=w244:dbl)
          n76 = Multiply(x=w232, y=w239) -> (x*y=w243:dbl)
        }
      }
      n77 = To Double Precision Float(number=w205) -> (double precision float=w204:dbl)
      n78 = Subtract(x=w209, y=w210) -> (x-y=w197:dbl)
      n79 = Subtract(x=w208, y=w211) -> (x-y=w196:dbl)
      n80 = Subtract(x=w207, y=w212) -> (x-y=w206:dbl)
    }
  }
  n81 = case "Accelerometer Read" shown="True" w47 {
    tunnel: w73 -> [_ w308]
    tunnel: w72 -> [_ w307]
    tunnel: w71 -> [_ w306]
    tunnel: w70 -> [_ w305]
    tunnel: w5 -> [_ w302]
    tunnel: [w271 w301] -> w39
    tunnel: "error in" -> [w271 w300]
    tunnel: w65 -> [_ w299]
    tunnel: w58 -> [_ w295]
    tunnel: w57 -> [_ w294]
    tunnel: w56 -> [_ w292]
    tunnel: [w272 w290] -> w55
    tunnel: [w272 w289] -> w54
    tunnel: [w272 w288] -> w53
    tunnel: [w270 w279] -> w51
    tunnel: w50 -> [_ w275]
    tunnel: [w270 w274] -> w37
    frame False {
      w272 = 0.0
      w270 = FALSE
    }
    frame True {
      w277 = 0.0 ("upper limit")
      w282 = 1.0 ("upper limit")
      n82 = case shown="False" w299 {
        tunnel: w302 -> [w351 w361]
        tunnel: [w355 w361] -> w304
        tunnel: [w352 TRUE] -> w303
        frame False {
          n83 = Build Array(u8 39 ("Data To Send")) -> (w359:u8[])
          n84 = call <vilib>:"WPI_I2CRead.vi"("I2CBytesToRead"=u8 1, "I2CRegister"=w359, "I2CDevRef"=w351) -> ("Data Out"=w356:u8[], "I2CDevRef"=w355:T6)  [unwired: 6 in, 1 out]
          n85 = Index Array(array=w356) -> (element=w354:u8)  [unwired: 1 in]
          n86 = And(x=w354, y=u8 8 ("Data To Send")) -> (x .and. y?=w353:u8)
          n87 = Not Equal To 0?(x=w353) -> (x != 0?=w352:bool)
        }
        frame True {
          # "Skip the status verification,\nassume data register will\nalways be ready.  Saves time\nby avoiding an I2C Read."
        }
      }
      n88 = case shown="True" w303 {
        tunnel: [w316 w327] -> w311
        tunnel: [w316 w326] -> w310
        tunnel: [w316 w325] -> w309
        tunnel: w308 -> [_ w324]
        tunnel: w304 -> [_ w323]
        tunnel: w300 -> [w313 w322]
        tunnel: [w312 w321] -> w301
        frame False {
          w316 = 0.0
          n89 = call <vilib>:"Error Cluster From Error Code.vi"("error in (no error)"=w313, "error message (\"\")"="Accel data register\nnot ready during \nread attempt" ("error message (\"\")"), "error code (0)"=259) -> ("error out"=w312:errorcluster)  [unwired: 6 in]
        }
        frame True {
          w317 = i16 -4 ("y")
          # "Accel data is left-justified so shift right 4 bits (arithmetically, to conserve sign)."
          n90 = case shown="0, Default" w324 {
            tunnel: [0.001 ("y") 0.002 ("y") 0.004 ("y") 0.012 ("y")] -> w328
            frame 0, Default {
              # "1 mG per LSB for 2 G range"
            }
            frame 1 {
              # "2 mG per LSB for 4 G range"
            }
            frame 2 {
              # "4 mG per LSB for 8 G range"
            }
            frame 3 {
              # "12 mG per LSB for 16 G range"
            }
          }
          n91 = Or(x=u8 128 ("Data To Send"), y=u8 40 ("Data To Send")) -> (x .or. y?=w341:u8)
          n92 = Build Array(w341) -> (w340:u8[])
          n93 = call <vilib>:"WPI_I2CRead.vi"("error in (no error)"=w322, "I2CBytesToRead"=u8 6, "I2CRegister"=w340, "I2CDevRef"=w323) -> ("error out"=w321:errorcluster, "Data Out"=w345:u8[])  [unwired: 5 in, 1 out]
          n94 = Index Array(array=w345) -> (element #1=w343:u8, element #2=w339:u8, element #3=w336:u8, element #4=w335:u8, element #5=w334:u8, element #6=w333:u8)  [unwired: 6 in]
          n95 = Join Numbers(hi=w339, lo=w343) -> ((hi.lo)=w344:u16)
          n96 = Join Numbers(hi=w335, lo=w336) -> ((hi.lo)=w337:u16)
          n97 = Join Numbers(hi=w333, lo=w334) -> ((hi.lo)=w338:u16)
          n98 = To Word Integer(number=w344) -> (16bit integer=w319:i16)
          n99 = To Word Integer(number=w337) -> (16bit integer=w320:i16)
          n100 = To Word Integer(number=w338) -> (16bit integer=w318:i16)
          n101 = Scale By Power Of 2(n=w317, x=w319) -> (x*2^n=w329:i16)
          n102 = Scale By Power Of 2(n=w317, x=w320) -> (x*2^n=w331:i16)
          n103 = Scale By Power Of 2(n=w317, x=w318) -> (x*2^n=w330:i16)
          n104 = Multiply(x=w329, y=w328) -> (x*y=w327:dbl)
          n105 = Multiply(x=w331, y=w328) -> (x*y=w326:dbl)
          n106 = Multiply(x=w330, y=w328) -> (x*y=w325:dbl)
        }
      }
      n107 = Multiply(x=w311, y=w307) -> (x*y=w298:dbl)
      n108 = Multiply(x=w310, y=w306) -> (x*y=w297:dbl)
      n109 = Multiply(x=w309, y=w305) -> (x*y=w296:dbl)
      n110 = Subtract(x=w292, y=1.0 ("x")) -> (x-y=w293:dbl)
      n111 = Subtract(x=w298, y=w295) -> (x-y=w290:dbl)
      n112 = Subtract(x=w297, y=w294) -> (x-y=w289:dbl)
      n113 = Subtract(x=w296, y=w293) -> (x-y=w288:dbl)
      n114 = Square(x=w290) -> (x^2=w287:dbl)
      n115 = Square(x=w289) -> (x^2=w286:dbl)
      n116 = Square(x=w288) -> (x^2=w285:dbl)
      n117 = Compound Arithmetic op=ADD(w287, w286, w285) -> (w284:dbl)
      n118 = Add(x=w275, y=w282) -> (x+y=w283:dbl)
      n119 = Subtract(x=w282, y=w275) -> (x-y=w281:dbl)
      n120 = Add(x=w275, y=w277) -> (x+y=w276:dbl)
      n121 = Subtract(x=w277, y=w275) -> (x-y=w278:dbl)
      n122 = Square Root(x=w284) -> (sqrt(x)=w273:dbl)
      n123 = In Range and Coerce(upper limit=w283, x=w273, lower limit=w281) -> (In Range?=w280:bool)  [unwired: 1 out]
      n124 = In Range and Coerce(upper limit=w276, x=w273, lower limit=w278) -> (In Range?=w274:bool)  [unwired: 1 out]
      n125 = Not(x=w280) -> (.not. x?=w279:bool)
    }
  }
  n126 = feedback #1(w78) -> (w79:dbl)
  n127 = feedback-in #1(w78) -> ()
  n128 = Subtract "dt (s)"(x=w78, y=w79) -> (x-y=w59:dbl)
  n129 = Equal To 0?(x=w19) -> (x = 0?=w83:bool)
  n130 = Unbundle By Name(w46) -> ("DevStatus"=w87:errorcluster)
  n131 = feedback #2(w29) -> (w32:dbl)
  n132 = feedback-in #2(w29) -> ()
  n133 = feedback #3(w24) -> (w27:dbl)
  n134 = feedback-in #3(w24) -> ()
  n135 = Add(x=w29, y=w32) -> (x+y=w31:dbl)
  n136 = feedback #4(w23) -> (w26:dbl)
  n137 = feedback-in #4(w23) -> ()
  n138 = Divide(x=w31, y=w22) -> (x/y=w30:dbl)
  n139 = Add(x=w24, y=w27) -> (x+y=w28:dbl)
  n140 = Bundle By Name(cluster="AdaIMUDevRef", "DevStatus"=w87, "Reset"=FALSE ("Fast")) -> (→"AdaIMUDevRef Out":T4)
  n141 = Divide(x=w28, y=w22) -> (x/y=w21:dbl)
  n142 = Add(x=w23, y=w26) -> (x+y=w25:dbl)
  n143 = Divide(x=w25, y=w22) -> (x/y=w20:dbl)
  n144 = case "Numerical Integration" shown="False" w83 {
    tunnel: w20 -> [w380 _]
    tunnel: [w379 w381] -> w82
    tunnel: w59 -> [w373 _]
    tunnel: w21 -> [w378 _]
    tunnel: w30 -> [w376 _]
    tunnel: [w375 w381] -> w81
    tunnel: [w374 w381] -> w80
    tunnel: w44 -> [w363 _]
    frame False {
      w366 = 0.0
      # "Accumulate displacements"
      n145 = Multiply(x=w373, y=w376) -> (x*y=w377:dbl)
      n146 = Multiply(x=w373, y=w378) -> (x*y=w370:dbl)
      n147 = Multiply(x=w373, y=w380) -> (x*y=w369:dbl)
      n148 = feedback #5(w366) -> (w371:dbl)
      n149 = Select(t=w366, s=w363, f=w371) -> (s? t:f=w372:dbl)
      n150 = Add(x=w377, y=w372) -> (x+y=w374:dbl)
      n151 = feedback-in #5(w374) -> ()
      n152 = feedback #6(w366) -> (w365:dbl)
      n153 = Select(t=w366, s=w363, f=w365) -> (s? t:f=w368:dbl)
      n154 = Add(x=w370, y=w368) -> (x+y=w375:dbl)
      n155 = feedback-in #6(w375) -> ()
      n156 = feedback #7(w366) -> (w364:dbl)
      n157 = Select(t=w366, s=w363, f=w364) -> (s? t:f=w367:dbl)
      n158 = Add(x=w369, y=w367) -> (x+y=w379:dbl)
      n159 = feedback-in #7(w379) -> ()
    }
    frame True {
      w381 = 0.0
      # "Avoid accumulating\ndegree displacements\nuntil calibrated\n(Once zero rate offsets\nare non-zero)."
    }
  }
  n160 = Bundle By Name(cluster=T1 {"Xaccel"=0.0, "Yaccel"=0.0, "Zaccel"=0.0, "Motion"=FALSE, "Threshold"=0.0, "FreeFall"=FALSE} ("input cluster"), "Xaccel"=w55, "Yaccel"=w54, "Zaccel"=w53, "Motion"=w51, "FreeFall"=w37) -> (→"Accel":T1)
  n161 = Bundle By Name(cluster=T2 {"Xmag"=0.0, "Ymag"=0.0, "Zmag"=0.0, "Anomaly"=FALSE}, "Xmag"=w62, "Ymag"=w61, "Zmag"=w60, "Anomaly"=w1) -> (→"Mag":T2)
  n162 = Merge Errors(w42, w39, w38) -> (→"error out":errorcluster)
  n163 = Bundle By Name(cluster=T3 {"Xrate"=0.0, "Yrate"=0.0, "Zrate"=0.0, "Xdeg"=0.0, "Ydeg"=0.0, "Zdeg"=0.0, "dt"=0.0} ("input cluster"), "Xdeg"=w80, "Ydeg"=w81, "Zdeg"=w82, "Xrate"=w29, "Yrate"=w24, "Zrate"=w23, "dt"=w59) -> (→"Gyro":T3)
